vi "Add Settings.vi"(0 "dsf refnum":T2, 1 "id":string, 7 "values":T1, 11 "error in (no error)":errorcluster) -> (4 "dsf refnum out":T2, 6 "plugin exists?":bool, 15 "error out":errorcluster)   [LabVIEW 2017, in "DSF Core.lvlib"]
uses:
  DSF Core.lvlib
  Public/Controls/DSF Config Data RefNum.ctl
  Public/Controls/DSF Settings Info.ctl
  Controls/DSF File Format/Internal.DSF Settings with ID.ctl
  Controls/DSF File Format/Internal.DSF Settings Info.ctl
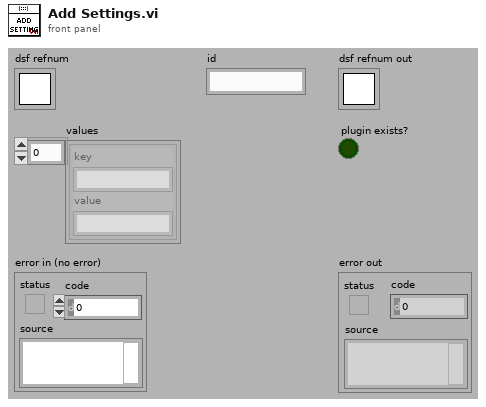
[diagram p1: front panel]
types:
  T1 = typedef "DSF Core.lvlib/DSF Settings Info.ctl" = cluster{"key":string, "value":string}[]
  T2 = typedef "DSF Core.lvlib/DSF Config Data RefNum.ctl" = refnum<k1>
  T3 = typedef "DSF Core.lvlib/Internal.DSF Settings with ID.ctl" = cluster{"id":string, "values":T4}
  T4 = typedef "DSF Core.lvlib/Internal.DSF Settings Info.ctl" = cluster{"key":string, "value":string}[]
  T5 = typedef "DSF Core.lvlib/DSF Configuration Reference.ctl" = refnum<data-value>
  T6 = typedef "DSF Core.lvlib/Internal.DSF Configuration.ctl" = cluster{"dsfversion":T7, "version":T7, "plugins":T8[], "groups":T11[], "transfers":T13[], "channels":T15[], "settings":T3[]}
  T7 = typedef "DSF Core.lvlib/DSF Version Info.ctl" = cluster{"major":u32, "minor":u32, "fix":u32, "build":string}
  T8 = typedef "DSF Core.lvlib/Internal.DSF Plugin with ID.ctl" = cluster{"id":string, "values":T9}
  T9 = typedef "DSF Core.lvlib/Internal.DSF Plugin Info.ctl" = cluster{"type":string, "timing":T10, "group ids":string[], "settings id":string}
  T10 = typedef "DSF Core.lvlib/DSF Timing Info.ctl" = cluster{"priority":u64, "decimation":u64, "offset":u64}
  T11 = typedef "DSF Core.lvlib/Internal.DSF Group with ID.ctl" = cluster{"id":string, "values":T12}
  T12 = typedef "DSF Core.lvlib/Internal.DSF Group Info.ctl" = cluster{"direction":i32, "timing":T10, "transfer ids":string[], "settings id":string}
  T13 = typedef "DSF Core.lvlib/Internal.DSF Transfer with ID.ctl" = cluster{"id":string, "values":T14}
  T14 = typedef "DSF Core.lvlib/Internal.DSF Transfer Info.ctl" = cluster{"byte order":i32, "channel ids":string[], "settings id":string}
  T15 = typedef "DSF Core.lvlib/Internal.DSF Channel with ID.ctl" = cluster{"id":string, "values":T16}
  T16 = typedef "DSF Core.lvlib/Internal.DSF Channel Info.ctl" = cluster{"count":u64, "buffer offset":u64, "data type":i32, "settings id":string}
  T17 = cluster{"dsf configuration":T6, "path":path, "dirty":bool}
  T18 = typedef "DSF Core.lvlib/DSF Config Data.ctl" = cluster{"dsf configuration":T6, "path":path, "dirty":bool}
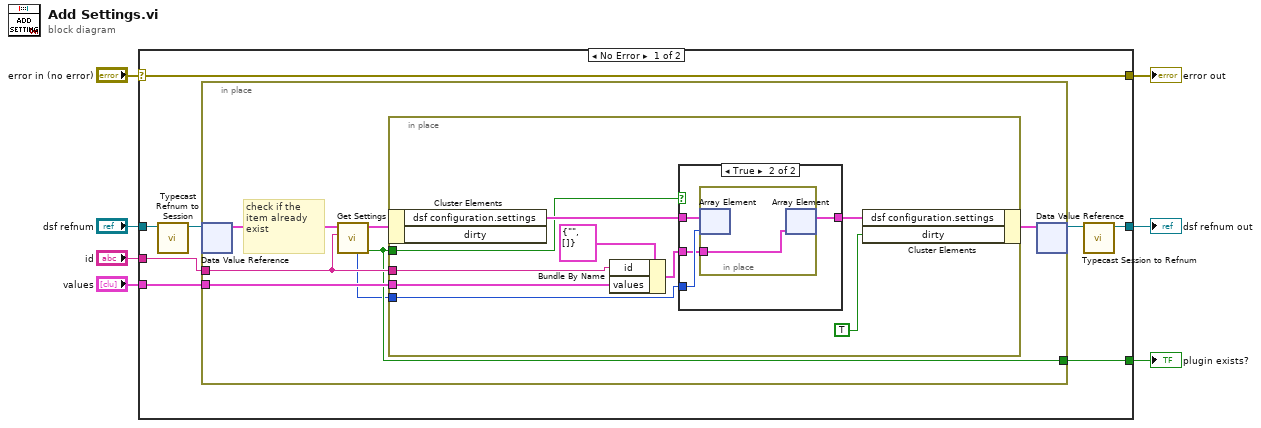
[diagram p0: block diagram]
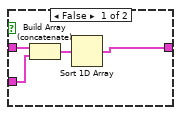
[diagram p2: hidden frame]
diagram:
  n1 = case shown="No Error" "error in (no error)" {
    selector: "error in (no error)" -> [w13 w42]
    tunnel: [w13 w42] -> w6
    tunnel: [w14 w41] -> w3
    tunnel: "dsf refnum" -> [w15 w41]
    tunnel: "id" -> [w12 _]
    tunnel: "values" -> [w11 _]
    tunnel: [w10 _] -> w1
    frame No Error {
      n2 = call "Typecast Refnum to Session.vi"("dsf refnum in"=w15) -> ("DSF Configuration Session out"=w9:T5)  [unwired: 10 out]
      n3 = in-place {
        in-place-border: w12 -> [w22]
        in-place-border: w11 -> [w20]
        in-place-border: [w19] -> w10
        # "check if the item already exist"
        n4 = in-place-dvr #1(w9) -> (w16:T17)  [unwired: 1 out]
        n5 = call "Get Settings.vi"("id"=w22, "DSF Configuration in"=w16) -> ("exists?"=w19:bool, "DSF Configuration out"=w21:T18, "index"=w18:i32)  [unwired: 6 in, 1 out]
        n6 = in-place {
          in-place-border: w22 -> [w30]
          in-place-border: w20 -> [w28]
          in-place-border: w19 -> [w27]
          in-place-border: w18 -> [w26]
          n7 = in-place-cluster #2(w21) -> ("dsf configuration.settings"=w31:T3[])  [unwired: 1 out]
          n8 = Bundle By Name(cluster=T3 {"id"="", "values"=[]} ("settings"), "id"=w30, "values"=w28) -> (w24:T3)
          n9 = case shown="True" w27 {
            tunnel: w31 -> [w35 w39]
            tunnel: [w34 w36] -> w29
            tunnel: w26 -> [_ w38]
            tunnel: w24 -> [w32 w37]
            frame False {
              n10 = Build Array (concatenate)(w35, w32) -> (w33:T3[])
              n11 = Sort 1D Array(array=w33) -> (sorted array=w34:T3[])
            }
            frame True {
              n12 = in-place {
                in-place-border: w37 -> [w40]
                n13 = in-place-array #3(w39, w38) -> ()  [unwired: 1 out]
                n14 = in-place-array #3(w40) -> (w36:T3[])  [unwired: 1 out]
              }
            }
          }
          n15 = in-place-cluster #2("dsf configuration.settings"=w29, "dirty"=TRUE) -> (w17:T18)
        }
        n16 = in-place-dvr #1(w17) -> (w8:T5)  [unwired: 1 out]
      }
      n17 = call "Typecast Session to Refnum.vi"("DSF Configuration Session in"=w8) -> ("dsf refnum out"=w14:T2)  [unwired: 10 out]
    }
    frame Error {
    }
  }
  "error out" <- w6
  "plugin exists?" <- w1
  "dsf refnum out" <- w3
